vi "Simple Queue.vi"() -> ()   [LabVIEW 2020]
doc: "VI创建了两个队列在并行循环间传输数据。如需从一个或多个数据源发送数据至一个数据接收器，且不损耗数据应使用队列。"
panel:
  out "数据 2":dbl(graph)
  out "数据 1":dbl(graph)
  in  "停止":bool
  # "概述：演示使用队列函数在并行循环间传输数据。\n操作步骤：\n运行VI。"
  # "程序框图上循环 1生成的数据通过队列传输至循环 2。循环 1内部会监控条件停止，并通过队列发送至循环 2。"
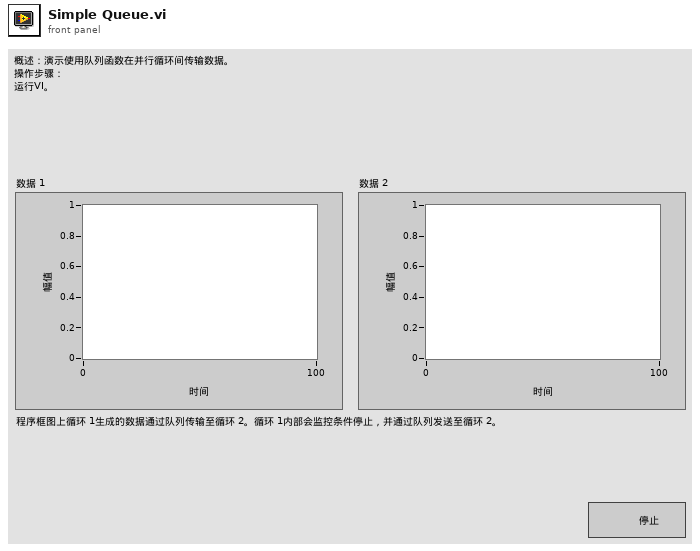
[diagram p1: front panel]
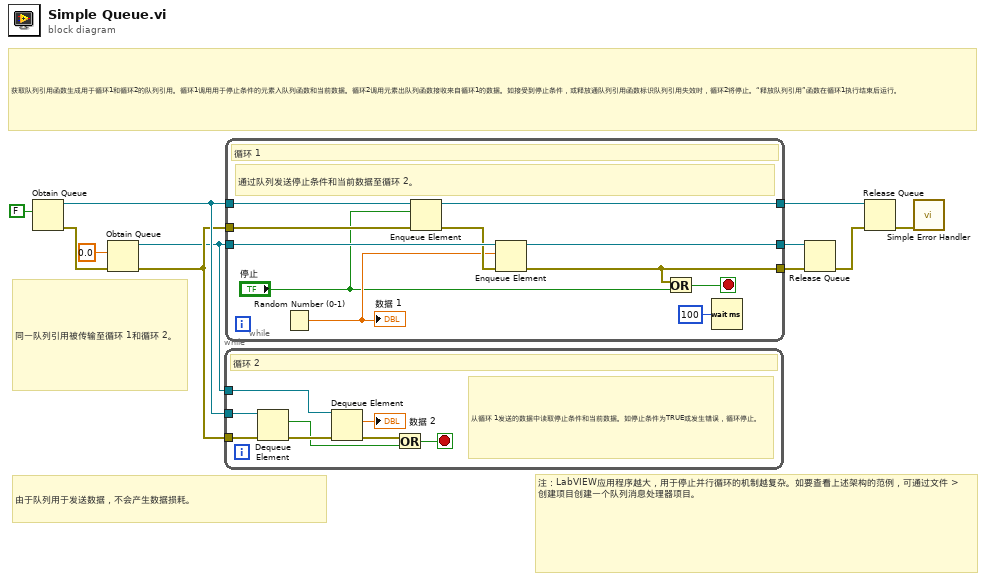
[diagram p0: block diagram]
diagram:
  # "由于队列用于发送数据，不会产生数据损耗。"
  # "注：LabVIEW应用程序越大，用于停止并行循环的机制越复杂。如要查看上述架构的范例，可通过文件 > 创建项目创建一个队列消息处理器项目。"
  # "同一队列引用被传输至循环 1和循环 2。"
  # "获取队列引用函数生成用于循环1和循环2的队列引用。循环1调用用于停止条件的元素入队列函数和当前数据。循环2调用元素出队列函数接收来自循环1的数据。如接受到停止条件，或释放通队列引用函数标识队列引用失效时，循环2将停止。“释放队列引用”函数在循环1执行结束后运行。"
  n1 = Obtain Queue(element data type=FALSE) -> (queue out=w11:refnum<queue>, error out=w9:errorcluster)  [unwired: 4 in, 1 out]
  n2 = Obtain Queue(element data type=0.0, error in (no error)=w9) -> (queue out=w1:refnum<queue>, error out=w2:errorcluster)  [unwired: 3 in, 1 out]
  n3 = while {
    tunnel: w11 -> [w18]
    tunnel: w2 -> [w19]
    tunnel: w1 -> [w16]
    stop <- w12 stop-if-true
    # "从循环 1发送的数据中读取停止条件和当前数据。如停止条件为TRUE或发生错误，循环停止。"
    # "循环 2"
    n4 = Dequeue Element(queue=w18, error in (no error)=w19) -> (element=w13:bool, error out=w17:errorcluster)  [unwired: 1 in, 2 out]
    n5 = Dequeue Element(queue=w16, error in (no error)=w17) -> (element=→"数据 2":dbl, error out=w14:errorcluster)  [unwired: 1 in, 2 out]
    n6 = Or(x=w14, y=w13) -> (x .or. y?=w12:bool)
  }
  n7 = while {
    tunnel: w11 -> [w29]
    tunnel: w2 -> [w28]
    tunnel: [w27] -> w4
    tunnel: w1 -> [w26]
    tunnel: [w24] -> w6
    tunnel: [w22] -> w7
    stop <- w20 stop-if-true
    # "通过队列发送停止条件和当前数据至循环 2。"
    # "循环 1"
    n8 = Random Number (0-1)() -> (number: 0 to 1=w23:dbl)
    "数据 1" <- w23
    n9 = Enqueue Element(queue=w29, element="停止", error in (no error)=w28) -> (queue out=w27:refnum<queue>, error out=w25:errorcluster)  [unwired: 1 in, 1 out]
    n10 = Enqueue Element(queue=w26, element=w23, error in (no error)=w25) -> (queue out=w24:refnum<queue>, error out=w22:errorcluster)  [unwired: 1 in, 1 out]
    n11 = Or(x=w22, y="停止") -> (x .or. y?=w20:bool)
    n12 = Wait (ms)(milliseconds to wait=u32 100) -> ()  [unwired: 1 out]
  }
  n13 = Release Queue(queue=w6, error in (no error)=w7) -> (error out=w5:errorcluster)  [unwired: 1 in, 2 out]
  n14 = Release Queue(queue=w4, error in (no error)=w5) -> (error out=w3:errorcluster)  [unwired: 1 in, 2 out]
  n15 = call <vilib>:"Simple Error Handler.vi"("error in (no error)"=w3) -> ()  [unwired: 4 in, 5 out]
